vi "Configure Clock Recovery Deemphasis.vi"(8 "error in (no error)":errorcluster, 10 "Clock Recovery De-emphasis (T: Enable)":bool=TRUE, 11 "VISA resource name":refnum<visa-resource-name>) -> (0 "error out":errorcluster, 3 "VISA resource name out":refnum<visa-resource-name>)   [LabVIEW 2020, in "Agilent 90000 Series.lvlib"]
doc: "Configures the settings specific to Recovered Clock Measurement."
uses:
  Agilent 90000 Series.lvlib
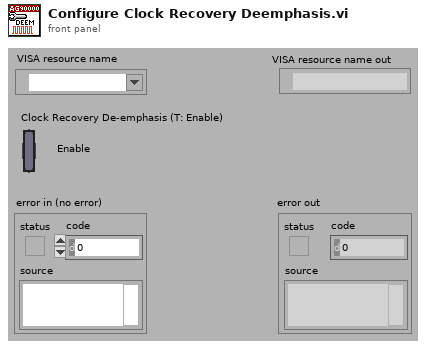
[diagram p1: front panel]
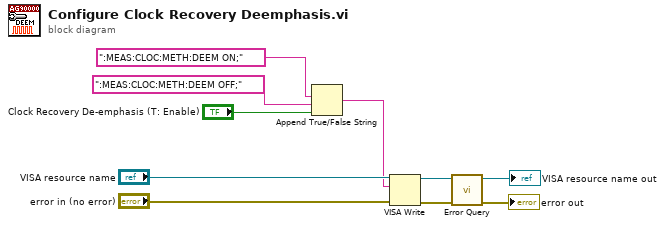
[diagram p0: block diagram]
diagram:
  n1 = Append True/False String(1:"Clock Recovery De-emphasis (T: Enable)", 2:":MEAS:CLOC:METH:DEEM OFF;" ("format string"), 3:":MEAS:CLOC:METH:DEEM ON;" ("format string")) -> (0:w2:string)  [unwired: 1 out]
  n2 = VISA Write(VISA resource name="VISA resource name", write buffer=w2, error in (no error)="error in (no error)") -> (VISA resource name out=w8:refnum<visa-resource-name>, error out=w7:errorcluster)  [unwired: 1 out]
  n3 = call "Error Query.vi"("error in (no error)"=w7, "VISA resource name"=w8) -> ("error out"=→"error out":errorcluster, "VISA resource name out"=→"VISA resource name out":refnum<visa-resource-name>)  [unwired: 8 out]
